vi "Real Spectrum Averaging.vi"(3 "reset averaging (T)":bool=TRUE, 4 "number of averages":u32=10 min=1, 5 "weighting mode":enum16{"Linear", "Exponential"}(ring), 6 "real spectrum":dbl[](array[numeric]) format="%.2f") -> (0 "error out":errorcluster, 1 "averages completed":dbl format="%.2f", 2 "averaged real spectrum":dbl[](array[numeric]) format="%.2f")   [LabVIEW 2017]
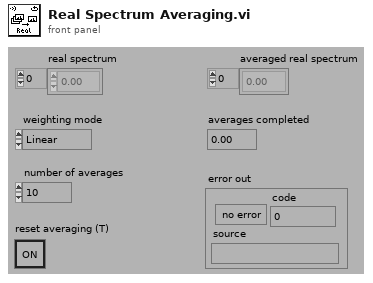
[diagram p1: front panel]
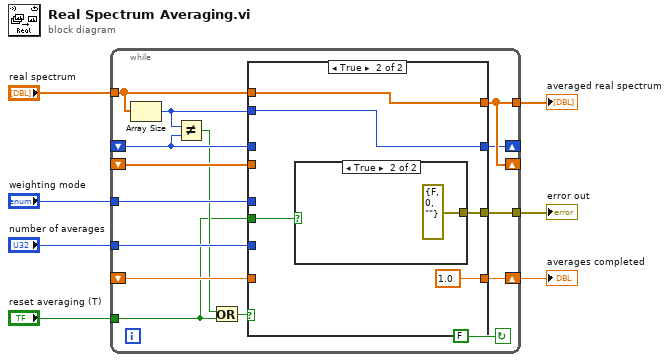
[diagram p0: block diagram]
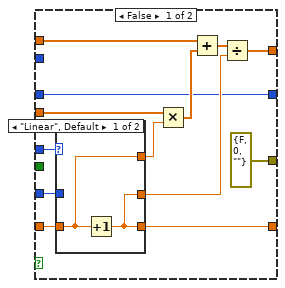
[diagram p2: hidden frame]
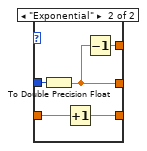
[diagram p3: hidden frame]
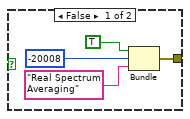
[diagram p4: hidden frame]
diagram:
  n1 = while {
    tunnel: [w11] -> w1
    shift-left: _ -> [w14]
    shift-right: [w16] -> _
    tunnel: "number of averages" -> [w17]
    tunnel: "weighting mode" -> [w18]
    tunnel: "real spectrum" -> [w15]
    shift-left: _ -> [w20]
    shift-right: [w21] -> w4
    shift-left: _ -> [w19]
    shift-right: [w22] -> _
    tunnel: [w22] -> w5
    tunnel: "reset averaging (T)" -> [w9]
    stop <- FALSE continue-if-true
    n2 = Array Size(array=w15) -> (size(s)=w13:i32)
    n3 = Not Equal?(x=w13, y=w14) -> (x != y?=w10:bool)
    n4 = Or(x=w10, y=w9) -> (x .or. y?=w12:bool)
    n5 = case shown="True" w12 {
      tunnel: [w32 w46] -> w22
      tunnel: [w27 1.0] -> w21
      tunnel: w20 -> [w30 _]
      tunnel: w19 -> [w35 _]
      tunnel: w15 -> [w31 w46]
      tunnel: w18 -> [w28 _]
      tunnel: w17 -> [w25 _]
      tunnel: [w24 w45] -> w16
      tunnel: w14 -> [w24 _]
      tunnel: w13 -> [_ w45]
      tunnel: [errorcluster {FALSE, 0, ""} w44] -> w11
      tunnel: w9 -> [_ w43]
      frame False {
        n6 = case shown="\"Linear\", Default" w28 {
          tunnel: w30 -> [w37 w41]
          tunnel: [w36 w42] -> w27
          tunnel: [w37 w38] -> w29
          tunnel: [w36 w39] -> w26
          tunnel: w25 -> [_ w40]
          frame "Linear", Default {
            n7 = Increment(x=w37) -> (x+1=w36:dbl)
          }
          frame "Exponential" {
            n8 = To Double Precision Float(number=w40) -> (double precision float=w39:dbl)
            n9 = Increment(x=w41) -> (x+1=w42:dbl)
            n10 = Decrement(x=w39) -> (x-1=w38:dbl)
          }
        }
        n11 = Multiply(x=w35, y=w29) -> (x*y=w34:dbl[])
        n12 = Add(x=w31, y=w34) -> (x+y=w33:dbl[])
        n13 = Divide(x=w33, y=w26) -> (x/y=w32:dbl[])
      }
      frame True {
        n14 = case shown="True" w43 {
          tunnel: [w48 errorcluster {FALSE, 0, ""}] -> w44
          frame False {
            n15 = Bundle(TRUE, -20008, "Real Spectrum Averaging") -> (w48:errorcluster)  [unwired: 1 in]
          }
          frame True {
          }
        }
      }
    }
  }
  "averaged real spectrum" <- w5
  "averages completed" <- w4
  "error out" <- w1
